vi "Write_States_ini.vi"(0 "Application_Directory":path, 11 "Error_In":errorcluster, 13 "State":T1=enum."Nature_of_the_Person") -> (15 "Error_Out":errorcluster)   [LabVIEW 2023]
doc: "This VI writes States to INI file."
uses:
  Controls/State.ctl
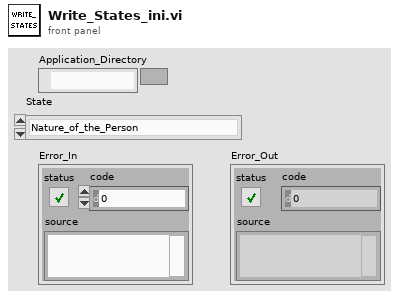
[diagram p1: front panel]
types:
  T1 = typedef "State.ctl" = enum16{"Close", "Password_Popup", "Start_Popup", "Wizard_Msg", "Get_Name_DoB", "Lucky_Number", "Q-1", "Q-2", "Q-3", "Nature_of_the_Person"}
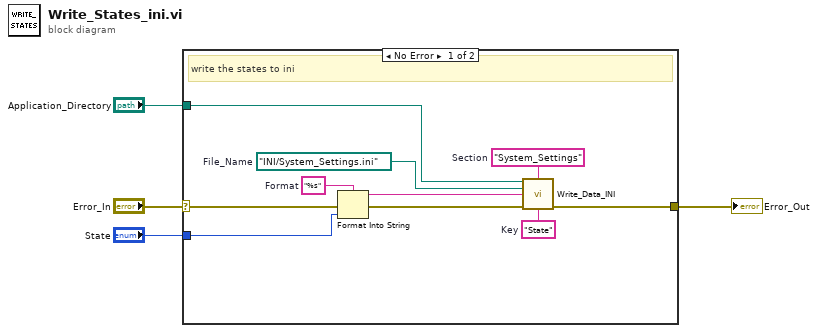
[diagram p0: block diagram]
diagram:
  n1 = case shown="No Error" "Error_In" {
    selector: "Error_In" -> [w14 w15]
    tunnel: "Application_Directory" -> [w9 _]
    tunnel: [w12 w15] -> w3
    tunnel: "State" -> [w5 _]
    frame No Error {
      w6 = "%s"  # Format
      w10 = "State"  # Key
      w11 = "System_Settings"  # Section
      w8 = path "INI/System_Settings.ini"  # File_Name
      # "write the states to ini"
      n2 = Format Into String(format string=w6, error in=w14, w5) -> (resulting string=w7:string, error out=w13:errorcluster)  [unwired: 1 in]
      n3 = call "Write_Data_INI.vi"("Application_Directory"=w9, "Section"=w11, "File_Name"=w8, "Data"=w7, "Error_In"=w13, "Key"=w10) -> ("Error_Out"=w12:errorcluster)  [unwired: 8 in, 1 out]
    }
    frame Error {
    }
  }
  "Error_Out" <- w3
